vi "Get RemIO Write Scaling Factor.vi"(8 "error in (no error)":errorcluster, 10 "11115 in":refnum<class "11115.lvclass">, 11 "Node Ptr In":T1 format="%.0x") -> (0 "error out":errorcluster, 1 "Scaling Factors":dbl[](array[numeric]), 2 "11115 out":refnum<class "11115.lvclass">, 3 "Node Ptr Out":T1 format="%.0x", 5 "Per Channel?":bool)   [LabVIEW 2017, in "Modules.lvlib" / "11115.lvclass"]
doc: "This VI Returns the scaling factors for REM IO Output Modules"
uses:
  11115.lvclass
  <vilib>/NI Veristand/Custom Device API/Custom Device Item Ref.ctl
  11115.lvclass/11115.ctl
  0dd47bb1-5308-42a9-8073-078de8be75cc.vi
  RemIO Module/Get RemIO Library Path.vi
  <vilib>/NI Veristand/Custom Device API/Custom Device API.lvlib
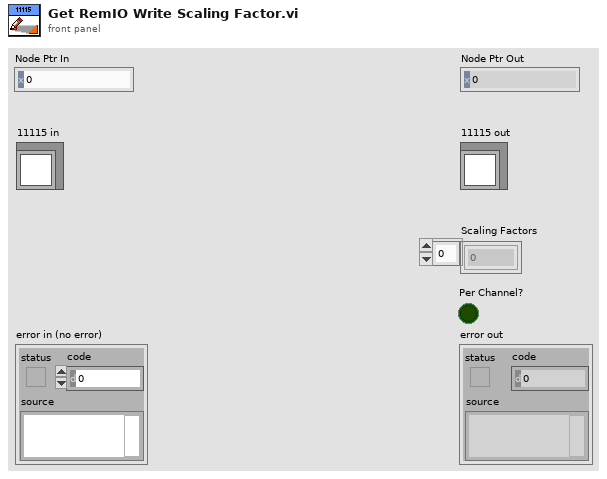
[diagram p1: front panel]
types:
  T1 = typedef "Custom Device API.lvlib/Custom Device Item Ref.ctl" = u64
  T2 = typedef "NI ECAT Remote IO.lvlib/channel number REM-11115.ctl" = u8
  T3 = typedef "NI ECAT Remote IO.lvlib/output range REM-11115.ctl" = u8
  T4 = cluster{"channel number":T2, "output range":T3}[]
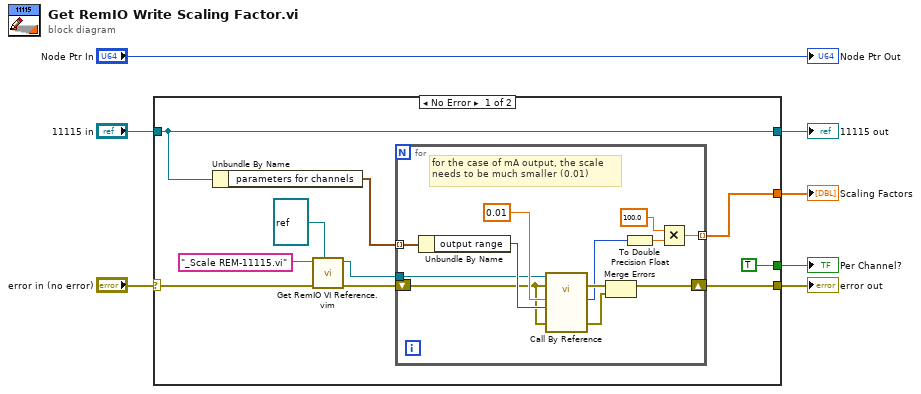
[diagram p0: block diagram]
diagram:
  n1 = case shown="No Error" "error in (no error)" {
    selector: "error in (no error)" -> [w12 w31]
    tunnel: [w15 w31] -> w6
    tunnel: [w16 w30] -> w4
    tunnel: "11115 in" -> [w16 w30]
    tunnel: [w13 _] -> w2
    tunnel: [TRUE _] -> w3
    frame No Error {
      n2 = Unbundle By Name(w16) -> ("parameters for channels"=w14:T4)
      n3 = call "Get RemIO VI Reference.vim"("name or relative path"="_Scale REM-11115.vi", "error in (no error)"=w12, "type specifier VI Refnum (for type only)"=refnum<vi> refnum) -> ("vi reference"=w8:refnum<vi>, "error out"=w11:errorcluster)  [unwired: 6 in]
      n4 = for {
        shift-right: [w20] -> w15
        shift-left: w11 -> [w19]
        tunnel: w14 -> [w29] mode=indexing
        tunnel: [w27] -> w13 mode=indexing
        tunnel: w8 -> [w18]
        # "for the case of mA output, the scale\nneeds to be much smaller (0.01)"
        n5 = Unbundle By Name(w29) -> ("output range"=w23:T3)
        n6 = call-by-ref "?"(reference=w18, error in=w19, 8:"error in (no error)"=w19, "output range"=w23, "scaled data"=0.01) -> (error out=w25:errorcluster, 0:"error out"=w21:errorcluster, "raw data"=w22:u16)  [unwired: 7 in, 1 out]
        n7 = Merge Errors(w25, w21) -> (w20:errorcluster)
        n8 = To Double Precision Float(number=w22) -> (double precision float=w28:dbl)
        n9 = Multiply(x=100.0, y=w28) -> (x*y=w27:dbl)
      }
    }
    frame Error {
    }
  }
  "error out" <- w6
  "11115 out" <- w4
  "Scaling Factors" <- w2
  "Per Channel?" <- w3
  "Node Ptr Out" <- "Node Ptr In"
